vi "2D Cartesian Coordinate Rotation (Scalar).vi"(9 "theta":dbl, 10 "y":dbl, 11 "x":dbl) -> (0 "error":i32, 2 "y out":dbl, 3 "x out":dbl)   [LabVIEW 2010, in "NI_AALPro.lvlib"]
doc: "Rotates a two-dimensional Cartesian coordinate in the counterclockwise direction. Wire data to the <B>X</B> input to determine the polymorphic instance to use or manually select the instance."
uses:
  NI_AALPro.lvlib
  lvanlys.dll
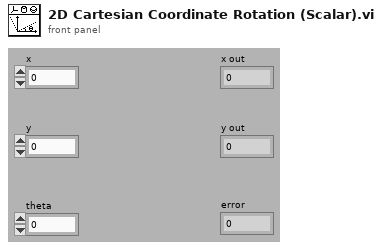
[diagram p1: front panel]
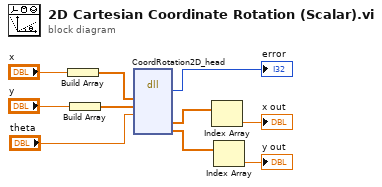
[diagram p0: block diagram]
diagram:
  n1 = Build Array("x") -> (w7:dbl[])
  n2 = Build Array("y") -> (w8:dbl[])
  n3 = dll-call lib="C:/Program Files/National Instruments/LabVIEW 2010/resource/lvanlys.*" fn="CoordRotation2D_head"("X"=w7, "Y"=w8, "theta"="theta") -> (→"error":i32, "Xout"=w5:dbl[], "Yout"=w3:dbl[])  [unwired: 8 in, 2 out]
  n4 = Index Array(array=w5) -> (element=→"x out":dbl)  [unwired: 1 in]
  n5 = Index Array(array=w3) -> (element=→"y out":dbl)  [unwired: 1 in]
